vi "multiFreqMultiSwitchMode.vi"(0 "步进电机串口":refnum<visa-resource-name>, 1 "单片机串口":refnum<visa-resource-name>, 2 "步进距离":dbl=5.0, 3 "步进频率":dbl=0.1) -> (4 "当前位置":dbl, 5 "当前频率":dbl, 6 "当前开关":dbl, 7 "参考信号":dbl[](array[numeric]), 8 "中频信号":dbl[](array[numeric]))   [LabVIEW 2018]
uses:
  <vilib>/Instr/_visa.llb/VISA Configure Serial Port (Instr).vi
  PCI8552B_32.dll
panel:
  out "待读取数据长度":i32
  out "频率变化次数":dbl
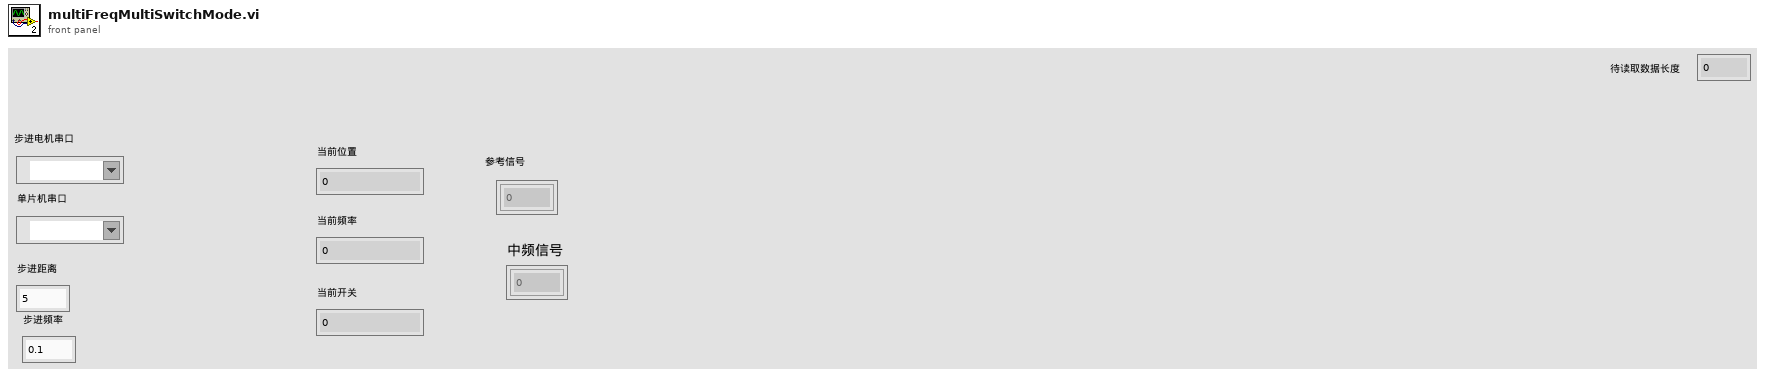
[diagram p1: front panel]
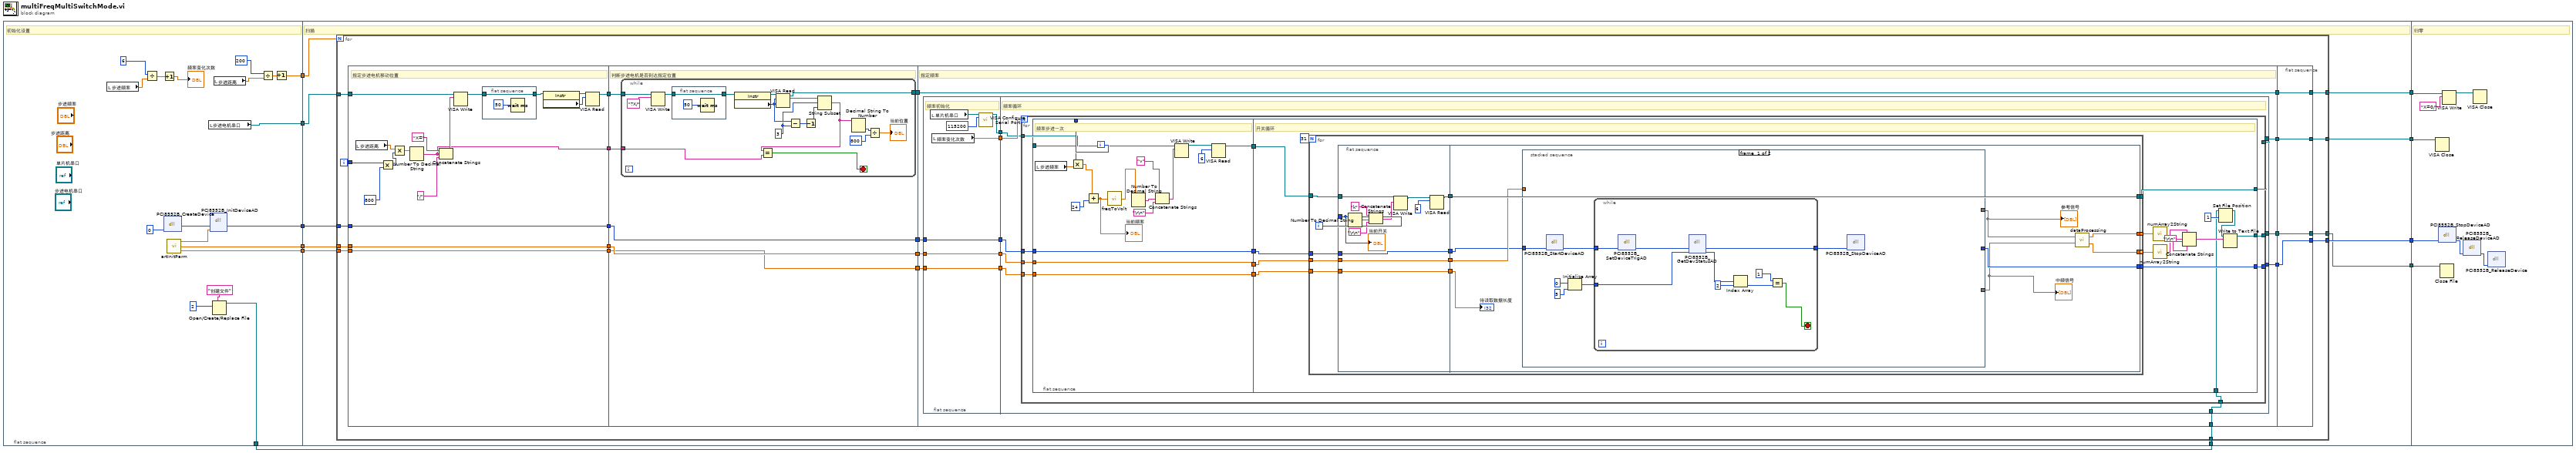
[diagram p0: block diagram]
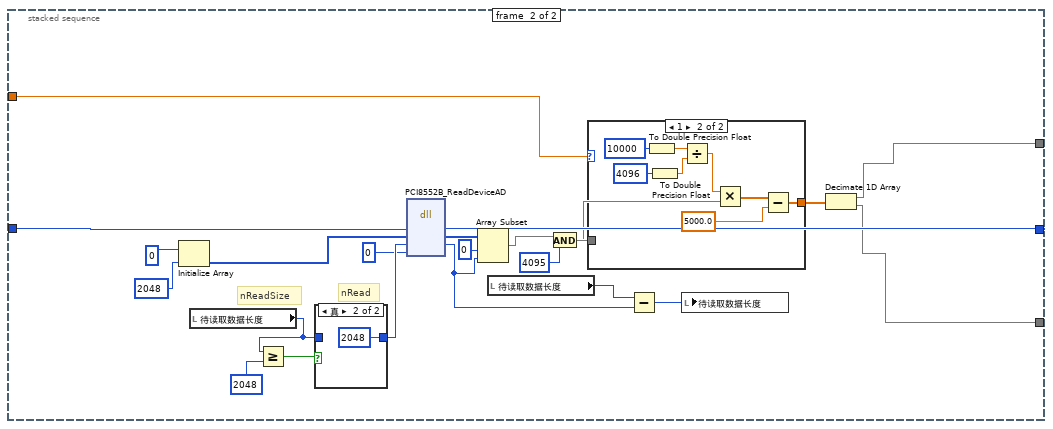
[diagram p2: hidden frame]
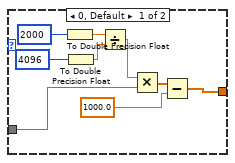
[diagram p3: hidden frame]
diagram:
  n1 = flat-sequence {
    tunnel: [w14] -> w10
    tunnel: [w11] -> w9
    tunnel: [w20] -> w6
    tunnel: [w19] -> w5
    tunnel: [w18] -> w4
    tunnel: [w15] -> w1
    tunnel: w10 -> [w38]
    tunnel: w9 -> [w37]
    tunnel: [w36] -> w8
    tunnel: [w35] -> w7
    tunnel: w6 -> [w34]
    tunnel: w5 -> [w33]
    tunnel: w4 -> [w32]
    tunnel: [w31] -> w3
    tunnel: [w30] -> w2
    tunnel: w1 -> [w29]
    tunnel: w8 -> [w283]
    tunnel: w7 -> [w282]
    tunnel: w3 -> [w279]
    tunnel: w2 -> [w278]
    frame #0 {
      # "初始化设置"
      n2 = local read "步进频率"() -> (w13:dbl)
      n3 = Divide(x=6, y=w13) -> (x/y=w25:dbl)
      n4 = Increment(x=w25) -> (x+1=→"频率变化次数":dbl)
      n5 = dll-call lib="PTH2|abs E\nPersonal File研究生学习202002-202007研一下学期work2020MMW Controllermmw_controllerPCI8552B_32" fn="PCI8552B_CreateDevice" label="CreateDevice"("DeviceLgcID"=0) -> ("返回类型"=w22:i32)  [unwired: 4 in, 2 out]
      n6 = call "artInitParm.vi"() -> ("待读取长度"=w18:dbl, "量程选择"=w19:dbl, "初始化参数"=w23:dbl[])
      n7 = local read "步进电机串口"() -> (w11:refnum<visa-resource-name>)
      n8 = dll-call lib="PTH2€abs E\nPersonal Fileç ”ç©¶ç”Ÿå­¦ä¹ 202002-202007ç ”ä¸€ä¸‹å­¦æœŸwork2020MMW Controllermmw_controllerPCI8552B_32.DLL" fn="PCI8552B_InitDeviceAD" label="InitDeviceAD"("hDevice"=w22, "pADPara"=w23) -> ("hDevice"=w20:i32)  [unwired: 5 in, 2 out]
      n9 = Open/Create/Replace File(prompt="创建文件", operation (0:open)=2) -> (refnum out=w15:refnum<file>)  [unwired: 4 in, 2 out]
      n10 = local read "步进距离"() -> (w12:dbl)
      n11 = Divide(x=200, y=w12) -> (x/y=w27:dbl)
      n12 = Increment(x=w27) -> (x+1=w14:dbl)
    }
    frame #1 {
      # "扫描"
      n13 = for {
        N: w38 -> [_]
        tunnel: w37 -> [w60]
        tunnel: [w55] -> w36
        tunnel: [w53] -> w35
        tunnel: w34 -> [w51]
        tunnel: w33 -> [w49]
        tunnel: w32 -> [w47]
        tunnel: [w42] -> w31
        tunnel: [w40] -> w30
        tunnel: w29 -> [w39]
        i -> [w61]
        n14 = flat-sequence "平铺式顺序结构" {
          tunnel: w61 -> [w62]
          tunnel: w60 -> [w75]
          tunnel: [w68] -> w59
          tunnel: [w66] -> w58
          tunnel: [w65] -> w52
          tunnel: w51 -> [w65]
          tunnel: [w64] -> w50
          tunnel: w49 -> [w64]
          tunnel: [w63] -> w48
          tunnel: w47 -> [w63]
          tunnel: w59 -> [w87]
          tunnel: w58 -> [w86]
          tunnel: [w85] -> w56
          tunnel: w52 -> [w84]
          tunnel: w50 -> [w83]
          tunnel: w48 -> [w82]
          tunnel: [w84] -> w46
          tunnel: [w83] -> w45
          tunnel: [w82] -> w44
          tunnel: [w119] -> w57
          tunnel: w56 -> [w119]
          tunnel: [w116] -> w54
          tunnel: w46 -> [w114]
          tunnel: w45 -> [w112]
          tunnel: w44 -> [w110]
          tunnel: [w109] -> w43
          tunnel: [w108] -> w41
          tunnel: w39 -> [w107]
          tunnel: w57 -> [w277]
          tunnel: [w277] -> w55
          tunnel: w54 -> [w276]
          tunnel: [w276] -> w53
          tunnel: w43 -> [w275]
          tunnel: [w275] -> w42
          tunnel: [w274] -> w40
          tunnel: w41 -> [w274]
          frame #0 {
            # "指定步进电机移动位置"
            n15 = local read "步进距离"() -> (w78:dbl)
            n16 = Multiply(x=w62, y=800) -> (x*y=w77:i32)
            n17 = Multiply(x=w78, y=w77) -> (x*y=w76:dbl)
            n18 = Number To Decimal String(number=w76) -> (decimal integer string=w66:string)  [unwired: 1 in]
            n19 = Concatenate Strings("X=", w66, "/") -> (w67:string)
            n20 = VISA Write(VISA resource name=w75, write buffer=w67) -> (VISA resource name out=w72:refnum<visa-resource-name>)  [unwired: 1 in, 2 out]
            n21 = flat-sequence {
              tunnel: w72 -> [w80]
              tunnel: [w80] -> w71
              frame #0 {
                n22 = Wait (ms)(milliseconds to wait=50) -> ()  [unwired: 1 out]
              }
            }
            n23 = property class="Instr"(reference=w71) -> (reference out=w70:refnum<visa-resource-name>, "Serial Settings:Number of Bytes at Serial Port"=w69:u32)  [unwired: 1 in, 1 out]
            n24 = VISA Read(VISA resource name=w70, byte count=w69) -> (VISA resource name out=w68:refnum<visa-resource-name>)  [unwired: 1 in, 3 out]
          }
          frame #1 {
            # "判断步进电机是否到达指定位置"
            n25 = while {
              tunnel: w87 -> [w104]
              tunnel: w86 -> [w94]
              tunnel: [w92] -> w85
              stop <- w93 stop-if-true
              w97 = 3
              n26 = VISA Write(VISA resource name=w104, write buffer="?X/") -> (VISA resource name out=w102:refnum<visa-resource-name>)  [unwired: 1 in, 2 out]
              n27 = flat-sequence {
                tunnel: w102 -> [w105]
                tunnel: [w105] -> w101
                frame #0 {
                  n28 = Wait (ms)(milliseconds to wait=50) -> ()  [unwired: 1 out]
                }
              }
              n29 = property class="Instr"(reference=w101) -> (reference out=w100:refnum<visa-resource-name>, "Serial Settings:Number of Bytes at Serial Port"=w98:u32)  [unwired: 1 in, 1 out]
              n30 = VISA Read(VISA resource name=w100, byte count=w98) -> (VISA resource name out=w92:refnum<visa-resource-name>, read buffer=w99:string)  [unwired: 1 in, 2 out]
              n31 = Subtract(x=w98, y=w97) -> (x-y=w96:u32)
              n32 = Decrement(x=w96) -> (x-1=w95:u32)
              n33 = String Subset(string=w99, offset (0)=w97, length (rest)=w95) -> (substring=w91:string)
              n34 = Equal?(x=w91, y=w94) -> (x = y?=w93:bool)
              n35 = Decimal String To Number(string=w91) -> (number=w90:i32)  [unwired: 2 in, 1 out]
              n36 = Divide(x=w90, y=800) -> (x/y=→"当前位置":dbl)
            }
          }
          frame #2 {
            # "指定频率"
            n37 = flat-sequence {
              tunnel: [w124] -> w118
              tunnel: [w123] -> w117
              tunnel: [w122] -> w115
              tunnel: w114 -> [w122]
              tunnel: [w121] -> w113
              tunnel: w112 -> [w121]
              tunnel: [w120] -> w111
              tunnel: w110 -> [w120]
              tunnel: w118 -> [w135]
              tunnel: w117 -> [w134]
              tunnel: [w133] -> w116
              tunnel: w115 -> [w132]
              tunnel: w113 -> [w131]
              tunnel: w111 -> [w130]
              tunnel: [w129] -> w109
              tunnel: [w128] -> w108
              tunnel: w107 -> [w127]
              frame #0 {
                # "频率初始化"
                n38 = local read "单片机串口"() -> (w125:refnum<visa-resource-name>)
                n39 = local read "频率变化次数"() -> (w124:dbl)
                n40 = call-poly "VISA Configure Serial Port"("VISA resource name"=w125, "baud rate (9600)"=115200) -> ("VISA resource name out"=w123:refnum<visa-resource-name>)  [unwired: 12 in, 1 out]
              }
              frame #1 {
                # "频率循环"
                n41 = for {
                  N: w135 -> [_]
                  tunnel: w134 -> [w147]
                  tunnel: [w145] -> w133
                  tunnel: w132 -> [w143]
                  tunnel: w131 -> [w141]
                  tunnel: w130 -> [w139]
                  tunnel: [w138] -> w129
                  tunnel: [w137] -> w128
                  tunnel: w127 -> [w136]
                  i -> [w148]
                  n42 = flat-sequence {
                    tunnel: w148 -> [w165]
                    tunnel: w147 -> [w161]
                    tunnel: [w157] -> w146
                    tunnel: [w151] -> w144
                    tunnel: w143 -> [w151]
                    tunnel: [w150] -> w142
                    tunnel: w141 -> [w150]
                    tunnel: [w149] -> w140
                    tunnel: w139 -> [w149]
                    tunnel: w146 -> [w181]
                    tunnel: [w180] -> w145
                    tunnel: w144 -> [w179]
                    tunnel: w142 -> [w178]
                    tunnel: w140 -> [w177]
                    tunnel: [w174] -> w138
                    tunnel: [w173] -> w137
                    tunnel: w136 -> [w170]
                    frame #0 {
                      # "频率步进一次"
                      n43 = local read "步进频率"() -> (w164:dbl)
                      n44 = Multiply(x=w165, y=w164) -> (x*y=w163:dbl)
                      n45 = Add(x=w163, y=24) -> (x+y=w152:dbl)
                      "当前频率" <- w152
                      n46 = call "freqToVolt.vi"("频率"=w152) -> ("电压"=w155:dbl)
                      n47 = Number To Decimal String(number=w155) -> (decimal integer string=w159:string)  [unwired: 1 in]
                      n48 = Concatenate Strings("v", w159, "\r\n") -> (w156:string)
                      n49 = VISA Write(VISA resource name=w161, write buffer=w156) -> (VISA resource name out=w154:refnum<visa-resource-name>)  [unwired: 1 in, 2 out]
                      n50 = VISA Read(VISA resource name=w154, byte count=6) -> (VISA resource name out=w157:refnum<visa-resource-name>)  [unwired: 1 in, 3 out]
                    }
                    frame #1 {
                      w172 = "\r\n"
                      # "开关循环"
                      n51 = for {
                        N: 31 -> [_]
                        tunnel: w181 -> [w195]
                        tunnel: [w194] -> w180
                        tunnel: w179 -> [w190]
                        tunnel: w178 -> [w188]
                        tunnel: w177 -> [w186]
                        tunnel: [w185] -> w174
                        tunnel: [w184] -> w169 mode=indexing
                        tunnel: [w183] -> w168 mode=indexing
                        i -> [w193]
                        n52 = flat-sequence {
                          tunnel: w195 -> [w207]
                          tunnel: w193 -> [w199]
                          tunnel: [w202] -> w192
                          tunnel: [w198] -> w191
                          tunnel: w190 -> [w198]
                          tunnel: [w197] -> w189
                          tunnel: w188 -> [w197]
                          tunnel: [w196] -> w187
                          tunnel: w186 -> [w196]
                          tunnel: [w216] -> w194
                          tunnel: w192 -> [w216]
                          tunnel: w191 -> [w214]
                          tunnel: w189 -> [w215]
                          tunnel: w187 -> [w213]
                          tunnel: [w212] -> w185
                          tunnel: [w211] -> w184
                          tunnel: [w210] -> w183
                          frame #0 {
                            n53 = Number To Decimal String(number=w199) -> (decimal integer string=w206:string)  [unwired: 1 in]
                            n54 = Concatenate Strings("k", w206, "\r\n") -> (w203:string)
                            n55 = VISA Write(VISA resource name=w207, write buffer=w203) -> (VISA resource name out=w201:refnum<visa-resource-name>)  [unwired: 1 in, 2 out]
                            n56 = VISA Read(VISA resource name=w201, byte count=6) -> (VISA resource name out=w202:refnum<visa-resource-name>)  [unwired: 1 in, 3 out]
                            "当前开关" <- w199
                          }
                          frame #1 {
                            n57 = stacked-sequence {
                              tunnel: w214 -> [w218 w249]
                              tunnel: [_ w253] -> w212
                              tunnel: w215 -> [_ w248]
                              tunnel: [_ w247] -> w208
                              tunnel: [_ w246] -> w209
                              frame #0 {
                                n58 = dll-call lib="PTH2€abs E\nPersonal Fileç ”ç©¶ç”Ÿå­¦ä¹ 202002-202007ç ”ä¸€ä¸‹å­¦æœŸwork2020MMW Controllermmw_controllerPCI8552B_32.DLL" fn="PCI8552B_StartDeviceAD" label="StartDeviceAD"("hDevice"=w218) -> ("hDevice"=w217:i32)  [unwired: 4 in, 2 out]
                                n59 = Initialize Array(0, 5) -> (w222:i32[])
                                n60 = while {
                                tunnel: w217 -> [w226]
                                tunnel: w222 -> [w231]
                                tunnel: [w224] -> w219
                                stop <- w223 stop-if-true
                                n61 = dll-call lib="PTH2€abs E\nPersonal Fileç ”ç©¶ç”Ÿå­¦ä¹ 202002-202007ç ”ä¸€ä¸‹å­¦æœŸwork2020MMW Controllermmw_controllerPCI8552B_32.DLL" fn="PCI8552B_SetDeviceTrigAD" label="SetDeviceTrigAD"("hDevice"=w226) -> ("hDevice"=w225:i32)  [unwired: 4 in, 2 out]
                                n62 = dll-call lib="PTH2€abs E\nPersonal Fileç ”ç©¶ç”Ÿå­¦ä¹ 202002-202007ç ”ä¸€ä¸‹å­¦æœŸwork2020MMW Controllermmw_controllerPCI8552B_32.DLL" fn="PCI8552B_GetDevStatusAD" label="GetDevStatusAD"("hDevice"=w225, "ADStatus"=w231) -> ("hDevice"=w224:i32, "ADStatus"=w227:i32[])  [unwired: 4 in, 2 out]
                                n63 = Index Array(array=w227, index=2) -> (element=w229:i32)
                                n64 = Equal?(x=1, y=w229) -> (x = y?=w223:bool)
                                }
                                n65 = dll-call lib="PTH2€abs E\nPersonal Fileç ”ç©¶ç”Ÿå­¦ä¹ 202002-202007ç ”ä¸€ä¸‹å­¦æœŸwork2020MMW Controllermmw_controllerPCI8552B_32.DLL" fn="PCI8552B_StopDeviceAD" label="StopDeviceAD"("hDevice"=w219) -> ()  [unwired: 5 in, 2 out]
                              }
                              frame #1 {
                                # "nReadSize"
                                # "nRead"
                                n66 = Initialize Array(u16 0 ("y"), 2048 ("y")) -> (w250:u16[])
                                n67 = local read "待读取数据长度"() -> (w243:i32)
                                n68 = Greater Or Equal?(x=w243, y=2048 ("millisecond multiple")) -> (x >= y?=w244:bool)
                                n69 = case shown="真" w244 {
                                tunnel: [w272 2048 ("millisecond multiple")] -> w240
                                tunnel: w243 -> [w272 _]
                                frame False {
                                }
                                frame True {
                                }
                                }
                                n70 = dll-call lib="PTH2€abs E\nPersonal Fileç ”ç©¶ç”Ÿå­¦ä¹ 202002-202007ç ”ä¸€ä¸‹å­¦æœŸwork2020MMW Controllermmw_controllerPCI8552B_32.DLL" fn="PCI8552B_ReadDeviceAD" label="ReadDeviceAD"("hDevice"=w249, "pADBuffer"=w250, "nReadSizeWords"=w240, "nRetSizeWords"=0) -> ("hDevice"=w253:i32, "pADBuffer"=w235:u16[], "nReadSizeWords"=w232:u32)  [unwired: 5 in, 2 out]
                                n71 = Array Subset(array=w235, index=0 ("索引"), length=w232) -> (w234:u16[])
                                n72 = local read "待读取数据长度"() -> (w242:i32)
                                n73 = And(x=w234, y=u16 4095) -> (x .and. y?=w238:u16[])
                                n74 = case shown="1" w248 {
                                tunnel: w238 -> [w261 w266]
                                tunnel: [w254 w265] -> w237
                                frame 0, Default {
                                n75 = To Double Precision Float(number=2000 ("x")) -> (double precision float=w257:dbl)
                                n76 = To Double Precision Float(number=4096) -> (double precision float=w256:dbl)
                                n77 = Divide(x=w257, y=w256) -> (x/y=w262:dbl)
                                n78 = Multiply(x=w262, y=w261) -> (x*y=w260:dbl[])
                                n79 = Subtract(x=w260, y=1000.0) -> (x-y=w254:dbl[])
                                }
                                frame 1 {
                                n80 = To Double Precision Float(number=10000 ("x")) -> (double precision float=w264:dbl)
                                n81 = To Double Precision Float(number=4096) -> (double precision float=w268:dbl)
                                n82 = Divide(x=w264, y=w268) -> (x/y=w271:dbl)
                                n83 = Multiply(x=w271, y=w266) -> (x*y=w270:dbl[])
                                n84 = Subtract(x=w270, y=5000.0) -> (x-y=w265:dbl[])
                                }
                                }
                                n85 = Subtract(x=w242, y=w232) -> (x-y=w241:u32)
                                n86 = local write "待读取数据长度"(w241) -> ()
                                n87 = Decimate 1D Array(w237) -> (w247:dbl[], w246:dbl[])
                              }
                            }
                            "中频信号" <- w209
                            "参考信号" <- w208
                            n88 = call "dataProcessing.vi"("中频信号"=w209, "参考信号"=w208) -> ("mean_Q"=w210:dbl, "mean_I"=w211:dbl)
                            "待读取数据长度" <- w213
                          }
                        }
                      }
                      n89 = call "numArray2String.vi"("输入数组"=w168) -> ("输出字符串"=w166:string)
                      n90 = call "numArray2String.vi"("输入数组"=w169) -> ("输出字符串"=w167:string)
                      n91 = Concatenate Strings(w166, w172, w167, w172) -> (w171:string)
                      n92 = Set File Position(refnum=w170, from (0:start)=1) -> (refnum out=w176:refnum<file>)  [unwired: 2 in, 1 out]
                      n93 = Write to Text File(file (use dialog)=w176, text=w171) -> (refnum out=w173:refnum<file>)  [unwired: 2 in, 2 out]
                    }
                  }
                }
              }
            }
          }
          frame #3 {
          }
        }
      }
    }
    frame #2 {
      # "归零"
      n94 = VISA Close(VISA resource name=w282) -> ()  [unwired: 1 in, 1 out]
      n95 = dll-call lib="PTH2€abs E\nPersonal Fileç ”ç©¶ç”Ÿå­¦ä¹ 202002-202007ç ”ä¸€ä¸‹å­¦æœŸwork2020MMW Controllermmw_controllerPCI8552B_32.DLL" fn="PCI8552B_StopDeviceAD" label="StopDeviceAD"("hDevice"=w279) -> ("hDevice"=w281:i32)  [unwired: 4 in, 2 out]
      n96 = Close File(refnum=w278) -> ()  [unwired: 1 in, 2 out]
      n97 = VISA Write(VISA resource name=w283, write buffer="X=0/") -> (VISA resource name out=w285:refnum<visa-resource-name>)  [unwired: 1 in, 2 out]
      n98 = dll-call lib="PTH2€abs E\nPersonal Fileç ”ç©¶ç”Ÿå­¦ä¹ 202002-202007ç ”ä¸€ä¸‹å­¦æœŸwork2020MMW Controllermmw_controllerPCI8552B_32.DLL" fn="PCI8552B_ReleaseDeviceAD" label="ReleaseDeviceAD"("hDevice"=w281) -> ("hDevice"=w280:i32)  [unwired: 4 in, 2 out]
      n99 = VISA Close(VISA resource name=w285) -> ()  [unwired: 1 in, 1 out]
      n100 = dll-call lib="PTH2€abs E\nPersonal Fileç ”ç©¶ç”Ÿå­¦ä¹ 202002-202007ç ”ä¸€ä¸‹å­¦æœŸwork2020MMW Controllermmw_controllerPCI8552B_32.DLL" fn="PCI8552B_ReleaseDevice" label="ReleaseDevice"("hDevice"=w280) -> ()  [unwired: 5 in, 2 out]
    }
  }
